vi "Handle Error Connected.vi"(8 "error in":errorcluster, 11 "server in":refnum<class "RT FlexRIO Server TCP.lvclass">) -> (0 "error out":errorcluster, 3 "server out":refnum<class "RT FlexRIO Server TCP.lvclass">)   [LabVIEW 2017, in "RT FlexRIO Server TCP.lvclass"]
uses:
  RT FlexRIO Server TCP.lvclass
  Public/State.ctl
  Properties/State_SET.vi
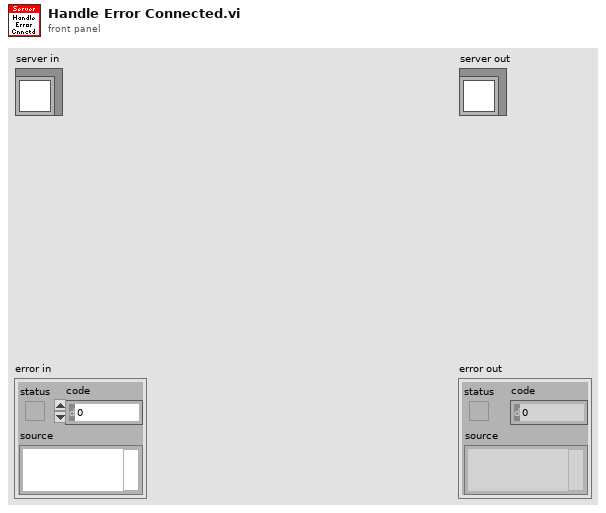
[diagram p1: front panel]
types:
  T1 = typedef "RT FlexRIO Server TCP.lvclass/State.ctl" = enum16{"started", "connected", "stopped"}
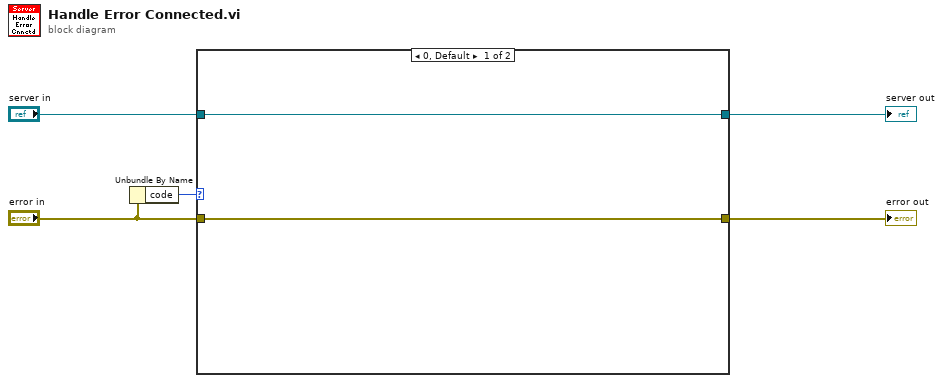
[diagram p0: block diagram]
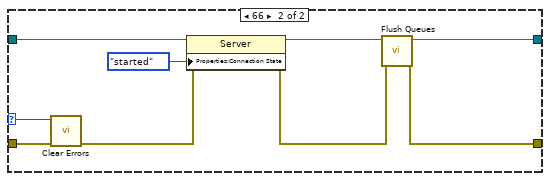
[diagram p2: hidden frame]
diagram:
  n1 = Unbundle By Name("error in") -> ("code"=w4:i32)
  n2 = case shown="0, Default" w4 {
    selector: w4 -> [_ w15]
    tunnel: "error in" -> [w7 w16]
    tunnel: "server in" -> [w6 w14]
    tunnel: [w7 w9] -> w2
    tunnel: [w6 w8] -> w1
    frame 0, Default {
    }
    frame 66 {
      n3 = call <vilib>:"Clear Errors.vi"("error in (no error)"=w16, "specific error code to clear (0: all)"=w15) -> ("error out"=w13:errorcluster)  [unwired: 4 in, 1 out]
      n4 = property class="Server"(reference=w14, error in=w13, "Properties:Connection State"=State."started" ("Connection State")) -> (reference out=w11:refnum<class "RT FlexRIO Server TCP.lvclass">, error out=w10:errorcluster)
      n5 = call "Flush Queues.vi"("error in"=w10, "server in"=w11) -> ("error out"=w9:errorcluster, "server out"=w8:refnum<class "RT FlexRIO Server TCP.lvclass">)  [unwired: 8 in]
    }
  }
  "error out" <- w2
  "server out" <- w1
